vi "Select Panel Object.vi"(6 "Select All Of Type":bool, 8 "Error In":errorcluster, 9 "Add To Selection":bool, 10 "Coords":T1, 11 "Pane Relief Main UI in":refnum<class "Pane Relief Main UI.lvclass">) -> (0 "Error Out":errorcluster, 3 "Pane Relief Main UI out":refnum<class "Pane Relief Main UI.lvclass">)   [LabVIEW 2017, in "Pane Relief Main UI.lvlib" / "Pane Relief Main UI.lvclass"]
uses:
  Pane Relief Main UI.lvclass
  <vilib>/Utility/miscctls.llb/LVPoint32TypeDef.ctl
  Pane Relief Main UI.lvclass/Pane Relief Main UI.ctl
  C/Program Files (x86)/National Instruments/LabVIEW 2017/user.lib/_OpenG.lib/array/array.llb/Remove Duplicates from 1D Array (I32)__ogtk.vi
  Panel Object/Panel Object.lvclass
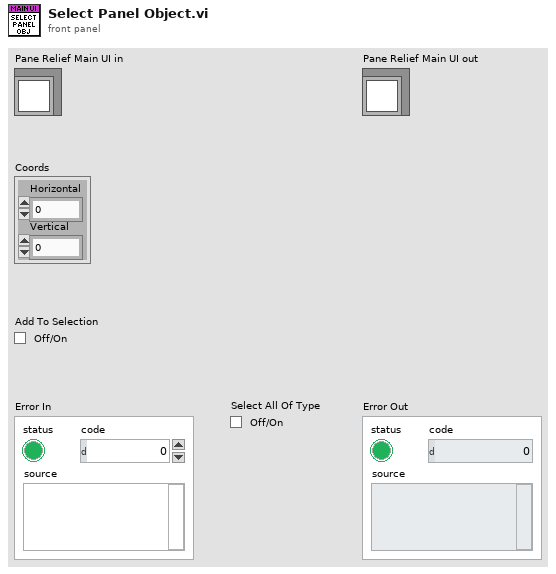
[diagram p1: front panel]
types:
  T1 = typedef "LVPoint32TypeDef.ctl" = cluster{"Horizontal":i32, "Vertical":i32}
  T2 = typedef "Point--Cluster.ctl" = cluster{"Horizontal":i32, "Vertical":i32}
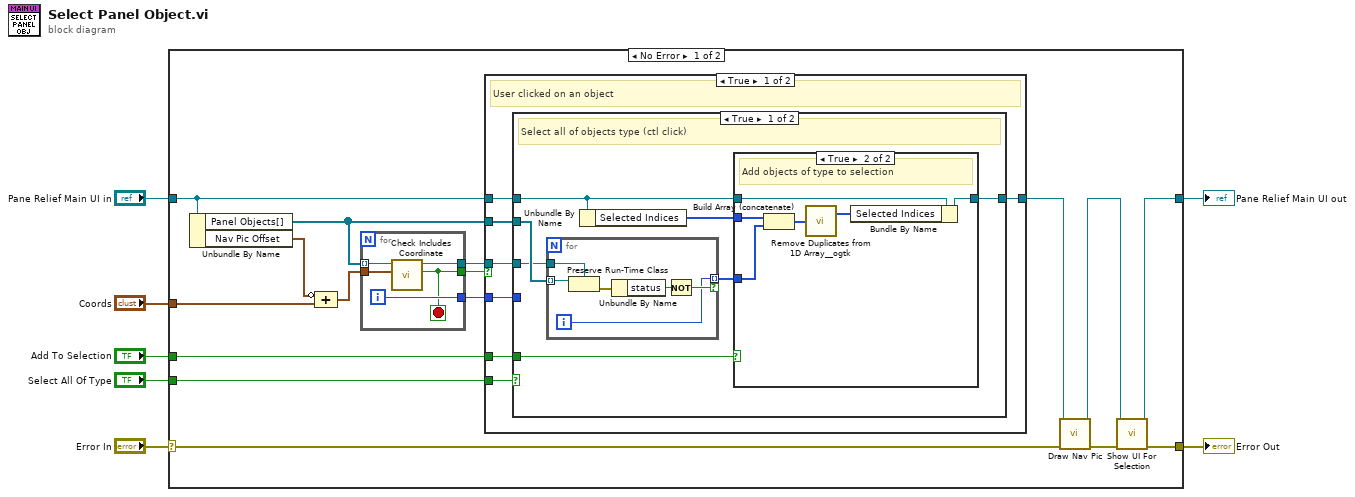
[diagram p0: block diagram]
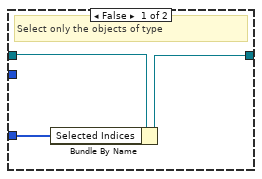
[diagram p2: hidden frame]
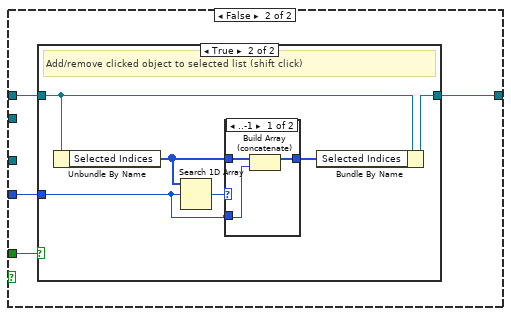
[diagram p3: hidden frame]
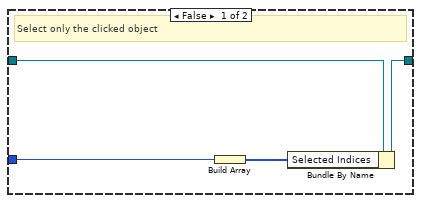
[diagram p4: hidden frame]
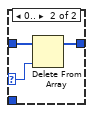
[diagram p5: hidden frame]
diagram:
  n1 = case shown="No Error" "Error In" {
    selector: "Error In" -> [w17 w80]
    tunnel: [w16 w80] -> w4
    tunnel: [w15 w79] -> w6
    tunnel: "Pane Relief Main UI in" -> [w12 w79]
    tunnel: "Coords" -> [w19 _]
    tunnel: "Add To Selection" -> [w11 _]
    tunnel: "Select All Of Type" -> [w8 _]
    frame No Error {
      n2 = Unbundle By Name(w12) -> ("Panel Objects[]"=w10:refnum<class "Panel Object.lvclass">[], "Nav Pic Offset"=w22:T2)
      n3 = Compound Arithmetic op=ADD(invert w22, w19) -> (w21:T2)
      n4 = for {
        tunnel: [w28] -> w9
        tunnel: [w24] -> w23
        tunnel: w10 -> [w27] mode=indexing
        tunnel: w21 -> [w26]
        tunnel: [w25] -> w20
        i -> [w25]
        stop <- w24 stop-if-true
        n5 = call-dynamic "Check Includes Coordinate.vi"("Coordinate"=w26, "Panel Object in"=w27) -> ("Included?"=w24:bool, "Panel Object out"=w28:refnum<class "Panel Object.lvclass">)  [unwired: 7 in, 1 out]
      }
      n6 = case shown="True" w23 {
        tunnel: w20 -> [w35 _]
        tunnel: [w32 w78] -> w13
        tunnel: w12 -> [w33 w78]
        tunnel: w11 -> [w34 _]
        tunnel: w10 -> [w31 _]
        tunnel: w9 -> [w30 _]
        tunnel: w8 -> [w29 _]
        frame True {
          # "User clicked on an object"
          n7 = case shown="True" w29 {
            tunnel: w35 -> [_ w61]
            tunnel: w34 -> [w42 w60]
            tunnel: w33 -> [w37 w59]
            tunnel: [w38 w58] -> w32
            tunnel: w31 -> [w41 _]
            tunnel: w30 -> [w40 _]
            frame True {
              # "Select all of objects type (ctl click)"
              n8 = for {
                tunnel: w41 -> [w46] mode=indexing
                tunnel: w40 -> [w45]
                tunnel: [w43] -> w39 mode=indexing if=w44
                i -> [w43]
                n9 = Preserve Run-Time Class(object in=w46, 2:w45) -> (error out=w48:errorcluster)  [unwired: 1 in, 1 out]
                n10 = Unbundle By Name(w48) -> ("status"=w47:bool)
                n11 = Not(x=w47) -> (.not. x?=w44:bool)
              }
              n12 = Unbundle By Name(w37) -> ("Selected Indices"=w36:i32[])
              n13 = case shown="True" w42 {
                tunnel: w37 -> [w50 w56]
                tunnel: w39 -> [w51 w54]
                tunnel: [w49 w57] -> w38
                tunnel: w36 -> [_ w55]
                frame False {
                  # "Select only the objects of type"
                  n14 = Bundle By Name(cluster=w50, "Selected Indices"=w51) -> (w49:refnum<class "Pane Relief Main UI.lvclass">)
                }
                frame True {
                  # "Add objects of type to selection"
                  n15 = Build Array (concatenate)(w55, w54) -> (w53:i32[])
                  n16 = call-poly "Remove Duplicates from 1D Array__ogtk.vi"("Input Array"=w53) -> ("Output Array"=w52:i32[])  [unwired: 1 out]
                  n17 = Bundle By Name(cluster=w56, "Selected Indices"=w52) -> (w57:refnum<class "Pane Relief Main UI.lvclass">)
                }
              }
            }
            frame False {
              n18 = case shown="True" w60 {
                tunnel: w61 -> [w65 w69]
                tunnel: w59 -> [w64 w67]
                tunnel: [w63 w66] -> w58
                frame False {
                  # "Select only the clicked object"
                  n19 = Build Array(w65) -> (w62:i32[])
                  n20 = Bundle By Name(cluster=w64, "Selected Indices"=w62) -> (w63:refnum<class "Pane Relief Main UI.lvclass">)
                }
                frame True {
                  # "Add/remove clicked object to selected list (shift click)"
                  n21 = Unbundle By Name(w67) -> ("Selected Indices"=w70:i32[])
                  n22 = Search 1D Array(1D array=w70, element=w69) -> (index of element=w71:i32)  [unwired: 1 in]
                  n23 = case shown="..-1" w71 {
                    selector: w71 -> [_ w76]
                    tunnel: w70 -> [w74 w77]
                    tunnel: [w72 w75] -> w68
                    tunnel: w69 -> [w73 _]
                    frame ..-1 {
                      n24 = Build Array (concatenate)(w74, w73) -> (w72:i32[])
                    }
                    frame 0.. {
                      n25 = Delete From Array(array=w77, index=w76) -> (array with subset deleted=w75:i32[])  [unwired: 1 in, 1 out]
                    }
                  }
                  n26 = Bundle By Name(cluster=w67, "Selected Indices"=w68) -> (w66:refnum<class "Pane Relief Main UI.lvclass">)
                }
              }
            }
          }
        }
        frame False {
          # "User did not click on an object"
        }
      }
      n27 = call-dynamic "Draw Nav Pic.vi"("Error In"=w17, "Pane Relief Main UI in"=w13) -> ("Error Out"=w18:errorcluster, "Pane Relief Main UI out"=w14:refnum<class "Pane Relief Main UI.lvclass">)  [unwired: 8 in]
      n28 = call-dynamic "Show UI For Selection.vi"("Error In"=w18, "Pane Relief Main UI in"=w14) -> ("Error Out"=w16:errorcluster, "Pane Relief Main UI out"=w15:refnum<class "Pane Relief Main UI.lvclass">)  [unwired: 8 in]
    }
    frame Error {
    }
  }
  "Pane Relief Main UI out" <- w6
  "Error Out" <- w4
